vi "sedSpectrometer_logEvent_MeasuredSpectrum.vi"(8 "error in (no error)":errorcluster, 11 "logevent_MeasuredSpectrum_Ctl":T1={"imageName"="", "wavelength[2048]"=array[2048 elements], "intensity[2048]"=array[2048 elements], "integrationTime"=0.0, "temperature"=0.0, "priority"=0}) -> (0 "error out":errorcluster, 2 "function return":i32, 3 "logevent_MeasuredSpectrum_Ctl out":T1)   [LabVIEW 2016, in "SALLV_sedSpectrometer.lvlib"]
doc: "int sedSpectrometer_shm_logEvent_MeasuredSpectrumLV(sedSpectrometer_logevent_MeasuredSpectrumLV *logevent_MeasuredSpectrum_Ctl );"
uses:
  SALLV_sedSpectrometer.lvlib
  DataTypes/logevent_MeasuredSpectrum.ctl
  SALLV_sedSpectrometer.so
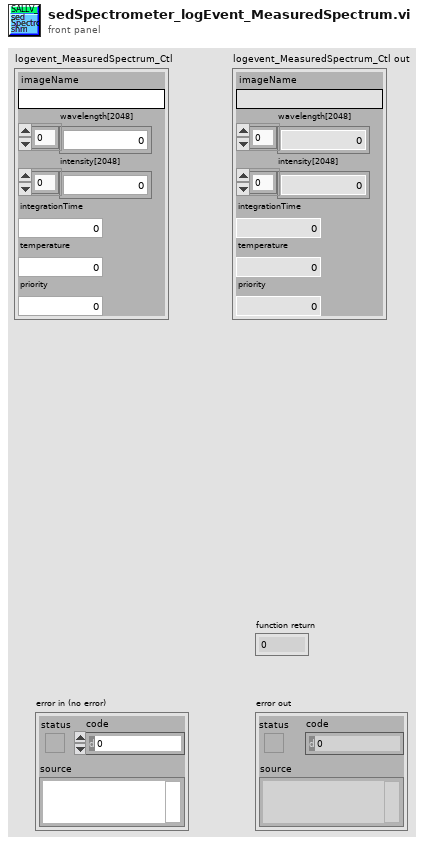
[diagram p1: front panel]
types:
  T1 = typedef "SALLV_sedSpectrometer.lvlib/logevent_MeasuredSpectrum.ctl" = cluster{"imageName":string, "wavelength[2048]":dbl[], "intensity[2048]":dbl[], "integrationTime":sgl, "temperature":dbl, "priority":i32}
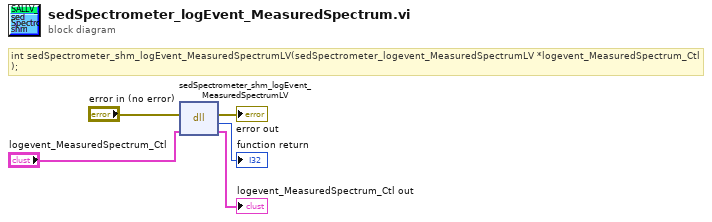
[diagram p0: block diagram]
diagram:
  # "int sedSpectrometer_shm_logEvent_MeasuredSpectrumLV(sedSpectrometer_logevent_MeasuredSpectrumLV *logevent_MeasuredSpectrum_Ctl );"
  n1 = dll-call lib="home/harini/TCS/sallv_sedSpectrometer/SALLV_sedSpectrometer.*" fn="sedSpectrometer_shm_logEvent_MeasuredSpectrumLV"(error in="error in (no error)", "logevent_MeasuredSpectrum_Ctl"="logevent_MeasuredSpectrum_Ctl") -> (error out=→"error out":errorcluster, →"function return":i32, "logevent_MeasuredSpectrum_Ctl"=→"logevent_MeasuredSpectrum_Ctl out":T1)  [unwired: 2 in, 1 out]
